vi "column bytes.vi"(8 "error in (no error)":errorcluster, 10 "iCol":i32, 11 "para0":u64) -> (0 "error out":errorcluster, 2 "column_bytes":i32, 3 "para0 out":u64)   [LabVIEW 2020, in "sqlite3.lvlib"]
uses:
  sqlite3.lvlib
  bin/sqlite3_64.dll
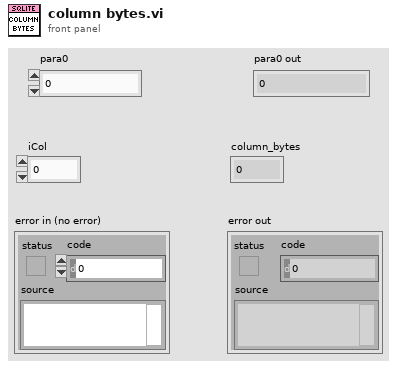
[diagram p1: front panel]
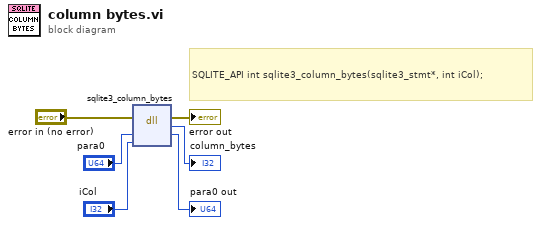
[diagram p0: block diagram]
diagram:
  # "SQLITE_API int sqlite3_column_bytes(sqlite3_stmt*, int iCol);"
  n1 = dll-call lib="D:/Project/Labview-Projects/database-configuration/externals/sqlite3/Source/bin/sqlite3_*.*" fn="sqlite3_column_bytes"(error in="error in (no error)", "para0"="para0", "iCol"="iCol") -> (error out=→"error out":errorcluster, "return type"=→"column_bytes":i32, "para0"=→"para0 out":u64)  [unwired: 3 in, 1 out]
